vi "New PI_2.vi"(0 "CtrlIndex":i32, 1 "LimitsArray":cluster{"Step":dbl, "Max":dbl, "Min":dbl}[](array[cluster]), 2 "FFinfo":T1(array[cluster]), 3 "PIinfo":T2(array[cluster]), 5 "CommandCluster":T4, 6 "Run?":bool, 7 "Feedback":dbl[](array[numeric]), 9 "CutoffArray":cluster{"MidCutoff":dbl, "CloseCutoff":dbl}[](array[cluster]), 11 "Stability In":T3, 12 "Tolerances":dbl[](array[numeric]), 13 "Controller?":bool, 14 "Ave Feedback":dbl[](array[numeric])) -> (4 "PIdata":dbl[](array[numeric]), 8 "Output":dbl, 10 "Stable?":bool, 15 "Stability Out":T3)   [LabVIEW 2013]
uses:
  TypeDef/Command Cluster.ctl
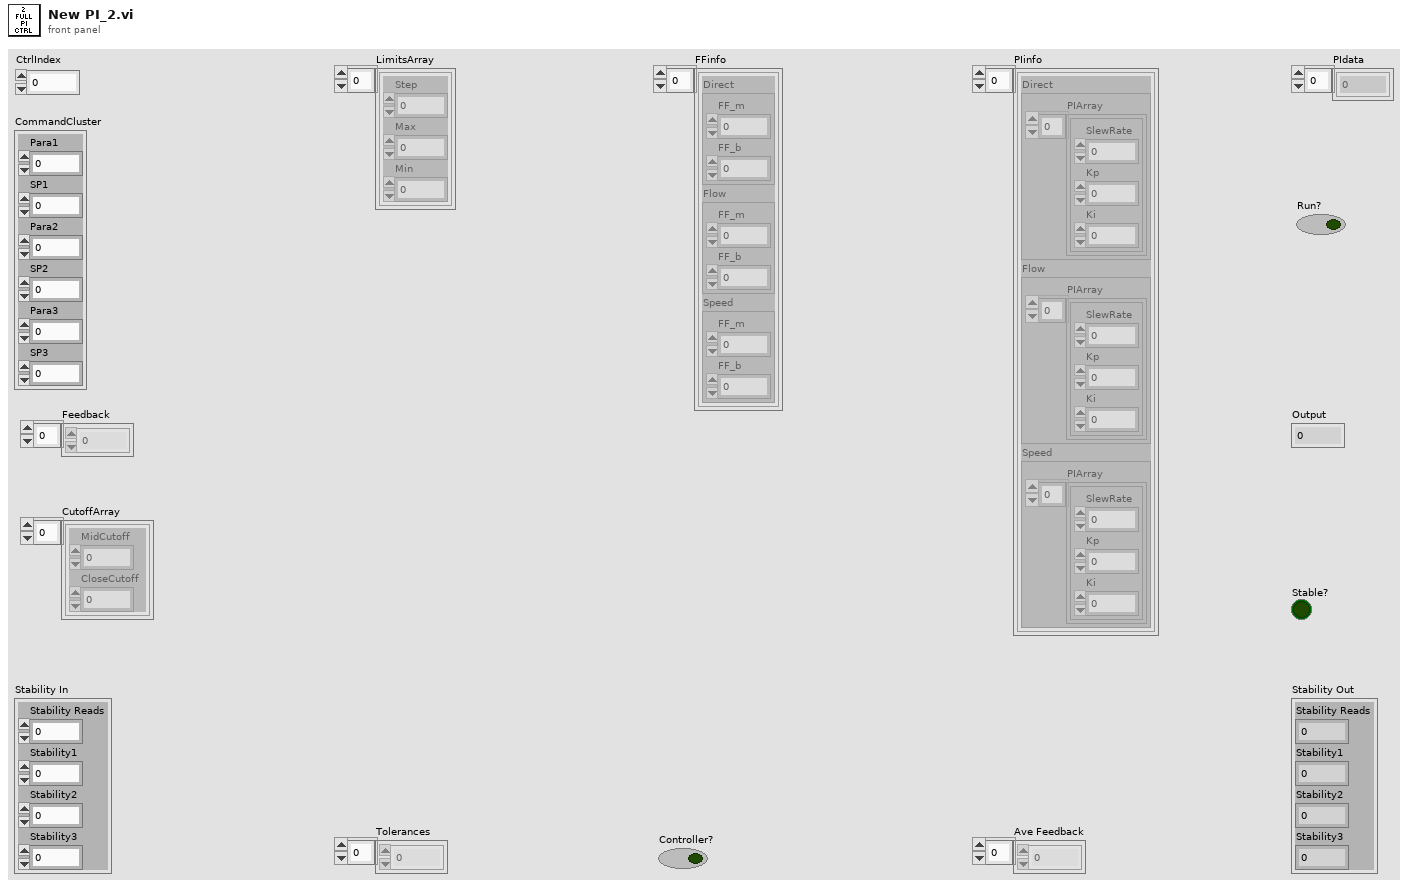
[diagram p1: front panel]
types:
  T1 = cluster{"Direct":cluster{"FF_m":dbl, "FF_b":dbl}, "Flow":cluster{"FF_m":dbl, "FF_b":dbl}, "Speed":cluster{"FF_m":dbl, "FF_b":dbl}}[]
  T2 = cluster{"Direct":cluster{"PIArray":cluster{"SlewRate":dbl, "Kp":dbl, "Ki":dbl}[]}, "Flow":cluster{"PIArray":cluster{"SlewRate":dbl, "Kp":dbl, "Ki":dbl}[]}, "Speed":cluster{"PIArray":cluster{"SlewRate":dbl, "Kp":dbl, "Ki":dbl}[]}}[]
  T3 = cluster{"Stability Reads":i32, "Stability1":i32, "Stability2":i32, "Stability3":i32}
  T4 = typedef "Command Cluster.ctl" = cluster{"Para1":i32, "SP1":dbl, "Para2":i32, "SP2":dbl, "Para3":i32, "SP3":dbl}
  T5 = cluster{"Direct":cluster{"FF_m":dbl, "FF_b":dbl}, "Flow":cluster{"FF_m":dbl, "FF_b":dbl}, "Speed":cluster{"FF_m":dbl, "FF_b":dbl}}
  T6 = cluster{"Direct":cluster{"PIArray":cluster{"SlewRate":dbl, "Kp":dbl, "Ki":dbl}[]}, "Flow":cluster{"PIArray":cluster{"SlewRate":dbl, "Kp":dbl, "Ki":dbl}[]}, "Speed":cluster{"PIArray":cluster{"SlewRate":dbl, "Kp":dbl, "Ki":dbl}[]}}
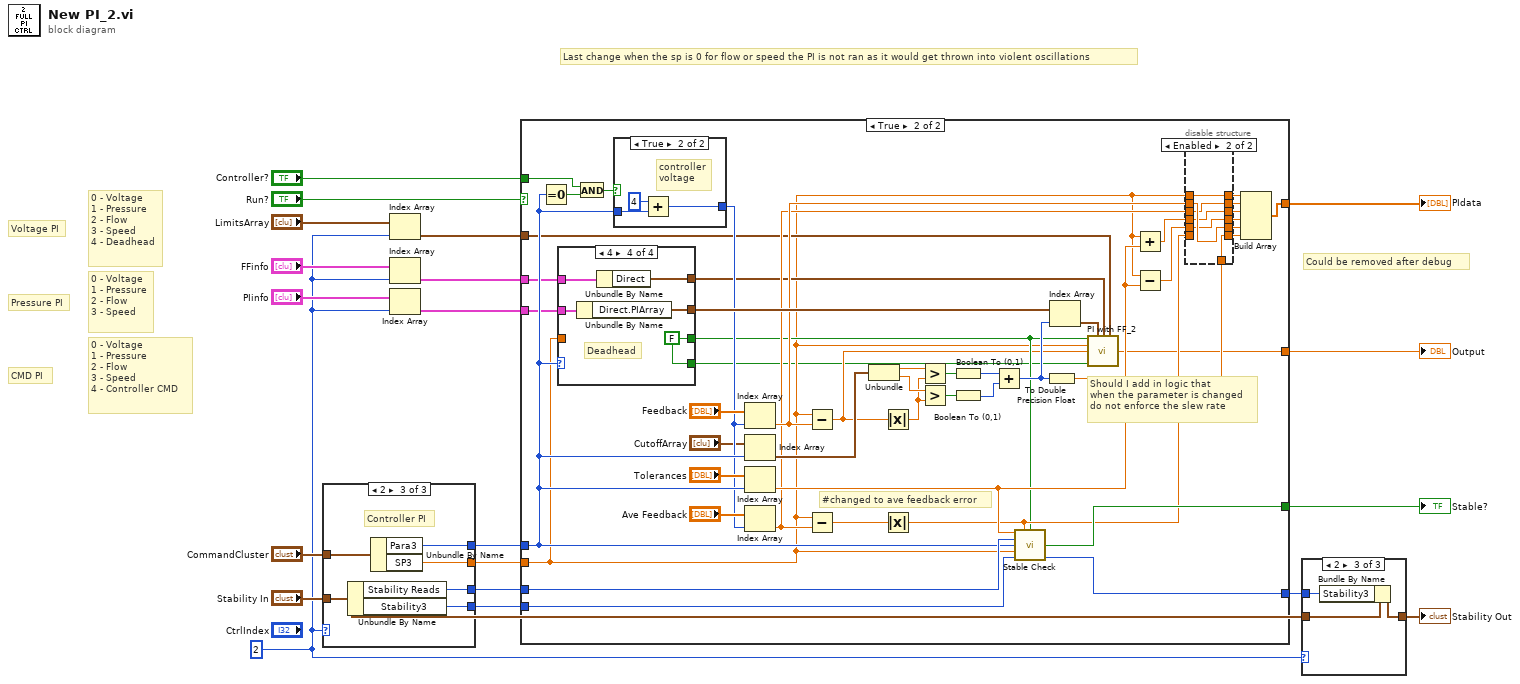
[diagram p0: block diagram]
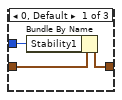
[diagram p2: hidden frame]
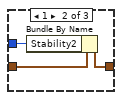
[diagram p3: hidden frame]
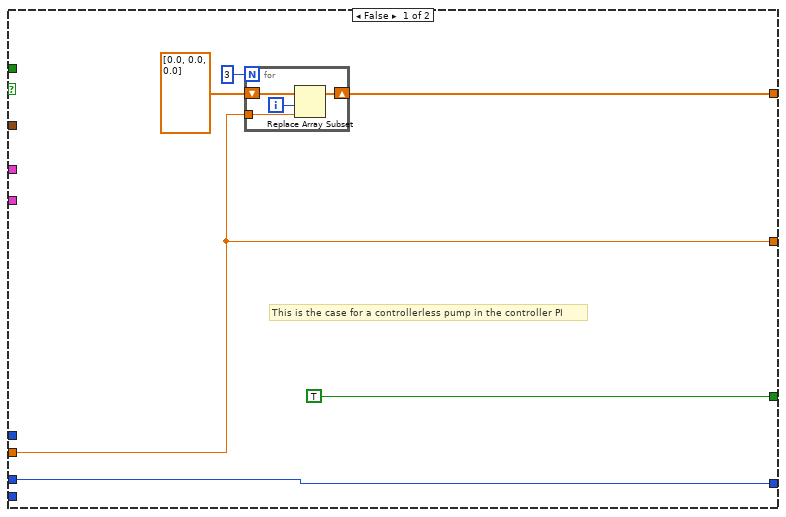
[diagram p4: hidden frame]
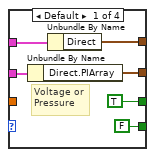
[diagram p7: hidden frame]
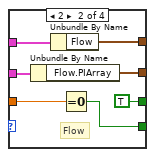
[diagram p8: hidden frame]
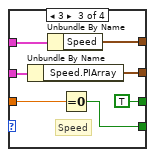
[diagram p9: hidden frame]
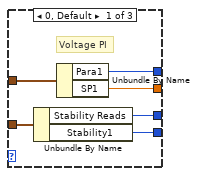
[diagram p10: hidden frame]
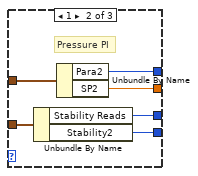
[diagram p11: hidden frame]
diagram:
  w4 = 2 ("CtrlIndex")
  # "Last change when the sp is 0 for flow or speed the PI is not ran as it would get thrown into violent oscillations"
  # "Could be removed after debug"
  # "CMD PI"
  # "Pressure PI"
  # "Voltage PI"
  # "0 - Voltage\n1 - Pressure\n2 - Flow\n3 - Speed\n4 - Controller CMD"
  # "0 - Voltage\n1 - Pressure\n2 - Flow\n3 - Speed"
  # "0 - Voltage\n1 - Pressure\n2 - Flow\n3 - Speed\n4 - Deadhead"
  n1 = case shown="2" w4 {
    tunnel: "Stability In" -> [w26 w32 w38]
    tunnel: [w24 w30 w36] -> w19
    tunnel: [w25 w31 w37] -> w18
    tunnel: "CommandCluster" -> [w23 w29 w35]
    tunnel: [w22 w28 w34] -> w3
    tunnel: [w21 w27 w33] -> w17
    frame 0, Default {
      # "Voltage PI"
      n2 = Unbundle By Name(w26) -> ("Stability Reads"=w24:i32, "Stability1"=w25:i32)
      n3 = Unbundle By Name(w23) -> ("Para1"=w22:i32, "SP1"=w21:dbl)
    }
    frame 1 {
      # "Pressure PI"
      n4 = Unbundle By Name(w32) -> ("Stability Reads"=w30:i32, "Stability2"=w31:i32)
      n5 = Unbundle By Name(w29) -> ("Para2"=w28:i32, "SP2"=w27:dbl)
    }
    frame 2 {
      # "Controller PI"
      n6 = Unbundle By Name(w38) -> ("Stability Reads"=w36:i32, "Stability3"=w37:i32)
      n7 = Unbundle By Name(w35) -> ("Para3"=w34:i32, "SP3"=w33:dbl)
    }
  }
  n8 = Index Array(array="LimitsArray", index=w4) -> (element=w9:cluster{"Step":dbl, "Max":dbl, "Min":dbl})
  n9 = Index Array(array="FFinfo", index=w4) -> (element=w5:T5)
  n10 = Index Array(array="PIinfo", index=w4) -> (element=w7:T6)
  n11 = case shown="True" "Run?" {
    tunnel: w19 -> [w43 w83]
    tunnel: w18 -> [_ w82]
    tunnel: w3 -> [_ w81]
    tunnel: w17 -> [w42 w52]
    tunnel: "Controller?" -> [_ w92]
    tunnel: [TRUE w71] -> w15
    tunnel: [w42 w49] -> w14
    tunnel: [w40 w91] -> w13
    tunnel: [w43 w84] -> w12
    tunnel: w9 -> [_ w53]
    tunnel: w7 -> [_ w79]
    tunnel: w5 -> [_ w77]
    frame False {
      # "This is the case for a controllerless pump in the controller PI"
      n12 = for {
        N: 3 -> [_]
        shift-right: [w47] -> w40
        shift-left: dbl[] [0.0, 0.0, 0.0] -> [w48]
        tunnel: w42 -> [w45]
        i -> [w46]
        n13 = Replace Array Subset(array=w48, new element=w45, index=w46) -> (w47:dbl[])
      }
    }
    frame True {
      # "#changed to ave feedback error"
      # "Should I add in logic that\nwhen the parameter is changed\ndo not enforce the slew rate"
      n14 = Equal To 0?(x=w81) -> (x = 0?=w95:bool)
      n15 = case shown="4" w81 {
        tunnel: [TRUE TRUE TRUE w133] -> w56
        tunnel: w79 -> [w117 w125 w132 w137]
        tunnel: [w116 w124 w131 w136] -> w78
        tunnel: w77 -> [w115 w123 w130 w135]
        tunnel: [w114 w122 w129 w134] -> w54
        tunnel: w52 -> [_ w121 w128 _]
        tunnel: [FALSE w120 w127 w133] -> w50
        frame Default {
          # "Voltage or\nPressure"
          n16 = Unbundle By Name(w117) -> ("Direct.PIArray"=w116:cluster{"SlewRate":dbl, "Kp":dbl, "Ki":dbl}[])
          n17 = Unbundle By Name(w115) -> ("Direct"=w114:cluster{"FF_m":dbl, "FF_b":dbl})
        }
        frame 2 {
          # "Flow"
          n18 = Unbundle By Name(w125) -> ("Flow.PIArray"=w124:cluster{"SlewRate":dbl, "Kp":dbl, "Ki":dbl}[])
          n19 = Unbundle By Name(w123) -> ("Flow"=w122:cluster{"FF_m":dbl, "FF_b":dbl})
          n20 = Equal To 0?(x=w121) -> (x = 0?=w120:bool)
        }
        frame 3 {
          # "Speed"
          n21 = Unbundle By Name(w132) -> ("Speed.PIArray"=w131:cluster{"SlewRate":dbl, "Kp":dbl, "Ki":dbl}[])
          n22 = Unbundle By Name(w130) -> ("Speed"=w129:cluster{"FF_m":dbl, "FF_b":dbl})
          n23 = Equal To 0?(x=w128) -> (x = 0?=w127:bool)
        }
        frame 4 {
          w133 = FALSE
          # "Deadhead"
          n24 = Unbundle By Name(w137) -> ("Direct.PIArray"=w136:cluster{"SlewRate":dbl, "Kp":dbl, "Ki":dbl}[])
          n25 = Unbundle By Name(w135) -> ("Direct"=w134:cluster{"FF_m":dbl, "FF_b":dbl})
        }
      }
      n26 = And(x=w92, y=w95) -> (x .and. y?=w94:bool)
      n27 = case shown="True" w94 {
        tunnel: w81 -> [w109 w112]
        tunnel: [w109 w110] -> w75
        frame False {
          # "pump\nvoltage"
        }
        frame True {
          # "controller\nvoltage"
          n28 = Add(x=4, y=w112) -> (x+y=w110:i32)
        }
      }
      n29 = Index Array(array="Feedback", index=w75) -> (element=w69:dbl)
      n30 = Index Array(array="CutoffArray", index=w81) -> (element=w80:cluster{"MidCutoff":dbl, "CloseCutoff":dbl})
      n31 = Index Array(array="Tolerances", index=w81) -> (element=w70:dbl)
      n32 = Index Array(array="Ave Feedback", index=w75) -> (element=w68:dbl)
      n33 = Subtract(x=w52, y=w69) -> (x-y=w51:dbl)
      n34 = Subtract(x=w52, y=w68) -> (x-y=w74:dbl)
      n35 = Unbundle(w80) -> ("MidCutoff"=w86:dbl, "CloseCutoff"=w85:dbl)
      n36 = Absolute Value(x=w51) -> (abs(x)=w73:dbl)
      n37 = Absolute Value(x=w74) -> (abs(x)=w65:dbl)
      n38 = Greater?(x=w86, y=w73) -> (0:w90:bool)
      n39 = Greater?(x=w85, y=w73) -> (0:w89:bool)
      n40 = Boolean To (0,1)(Boolean=w90) -> (0, 1=w88:i16)
      n41 = Boolean To (0,1)(Boolean=w89) -> (0, 1=w87:i16)
      n42 = Add(x=w88, y=w87) -> (x+y=w58:i16)
      n43 = call "Stable Check.vi"("Tolerance"=w70, "AbsError"=w65, "PI Running?"=w56, "ReqReads"=w83, "Parameter"=w81, "Setpoint"=w52, "StabilityCount In"=w82) -> ("Stable?"=w71:bool, "StabilityCount Out"=w84:i32)  [unwired: 6 in, 1 out]
      n44 = To Double Precision Float(number=w58) -> (double precision float=w57:dbl)
      n45 = Index Array(array=w78, index=w58) -> (element=w55:cluster{"SlewRate":dbl, "Kp":dbl, "Ki":dbl})
      n46 = call "PI with FF_2.vi"("Run PI?"=w56, "PIcluster"=w55, "FFcluster"=w54, "LimitCluster"=w53, "SP"=w52, "Error"=w51, "RevCtrlZero"=w50) -> ("Output"=w49:dbl)  [unwired: 7 in, 1 out]
      n47 = Add(x=w52, y=w70) -> (x+y=w67:dbl)
      n48 = Subtract(x=w52, y=w70) -> (x-y=w66:dbl)
      n49 = disable-structure shown="Enabled" {
        disable-tunnel: w52 -> [w102 w108]
        disable-tunnel: w69 -> [w101 w106]
        disable-tunnel: w68 -> [w100 w103]
        disable-tunnel: w67 -> [w99 w104]
        disable-tunnel: w66 -> [w98 w105]
        disable-tunnel: w65 -> [w97 _]
        disable-tunnel: [w102 w108] -> w64
        disable-tunnel: [w101 w103] -> w63
        disable-tunnel: [w100 w104] -> w62
        disable-tunnel: [w99 w105] -> w61
        disable-tunnel: [w98 w106] -> w60
        disable-tunnel: [w97 w107] -> w59
        disable-tunnel: w57 -> [_ w107]
        frame Disabled {
        }
        frame Enabled {
        }
      }
      n50 = Build Array(w64, w63, w62, w61, w60, w59) -> (w91:dbl[])
    }
  }
  "Stable?" <- w15
  "Output" <- w14
  "PIdata" <- w13
  n51 = case shown="2" w4 {
    tunnel: "Stability In" -> [w139 w142 w145]
    tunnel: [w138 w141 w144] -> w16
    tunnel: w12 -> [w140 w143 w146]
    frame 0, Default {
      n52 = Bundle By Name(cluster=w139, "Stability1"=w140) -> (w138:T3)
    }
    frame 1 {
      n53 = Bundle By Name(cluster=w142, "Stability2"=w143) -> (w141:T3)
    }
    frame 2 {
      n54 = Bundle By Name(cluster=w145, "Stability3"=w146) -> (w144:T3)
    }
  }
  "Stability Out" <- w16
